vi "Load Config.vi"(10 "Cluster":T1, 11 "Process":bool) -> ()   [LabVIEW 2016]
uses:
  <vilib>/Utility/config.llb/Read Key (Double).vi
  <vilib>/Utility/config.llb/Read Key (Boolean).vi
  <vilib>/Utility/config.llb/NI_LVConfig.lvlib
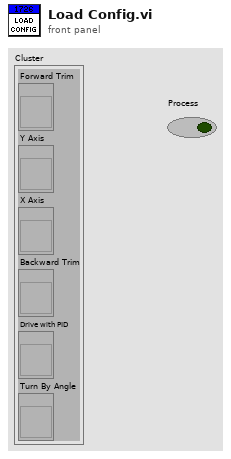
[diagram p1: front panel]
types:
  T1 = cluster{"Forward Trim":refnum<vi>, "Y Axis":refnum<vi>, "X Axis":refnum<vi>, "Backward Trim":refnum<vi>, "Drive with PID":refnum<vi>, "Turn By Angle":refnum<vi>}
  T2 = typedef "NI_LVConfig.lvlib/Config Data RefNum.ctl" = refnum<k1>
  T3 = cluster{"value":dbl, "value":dbl, "value":dbl, "value":bool}
  T4 = cluster{"value":dbl, dbl[], "value":dbl, "value":dbl}
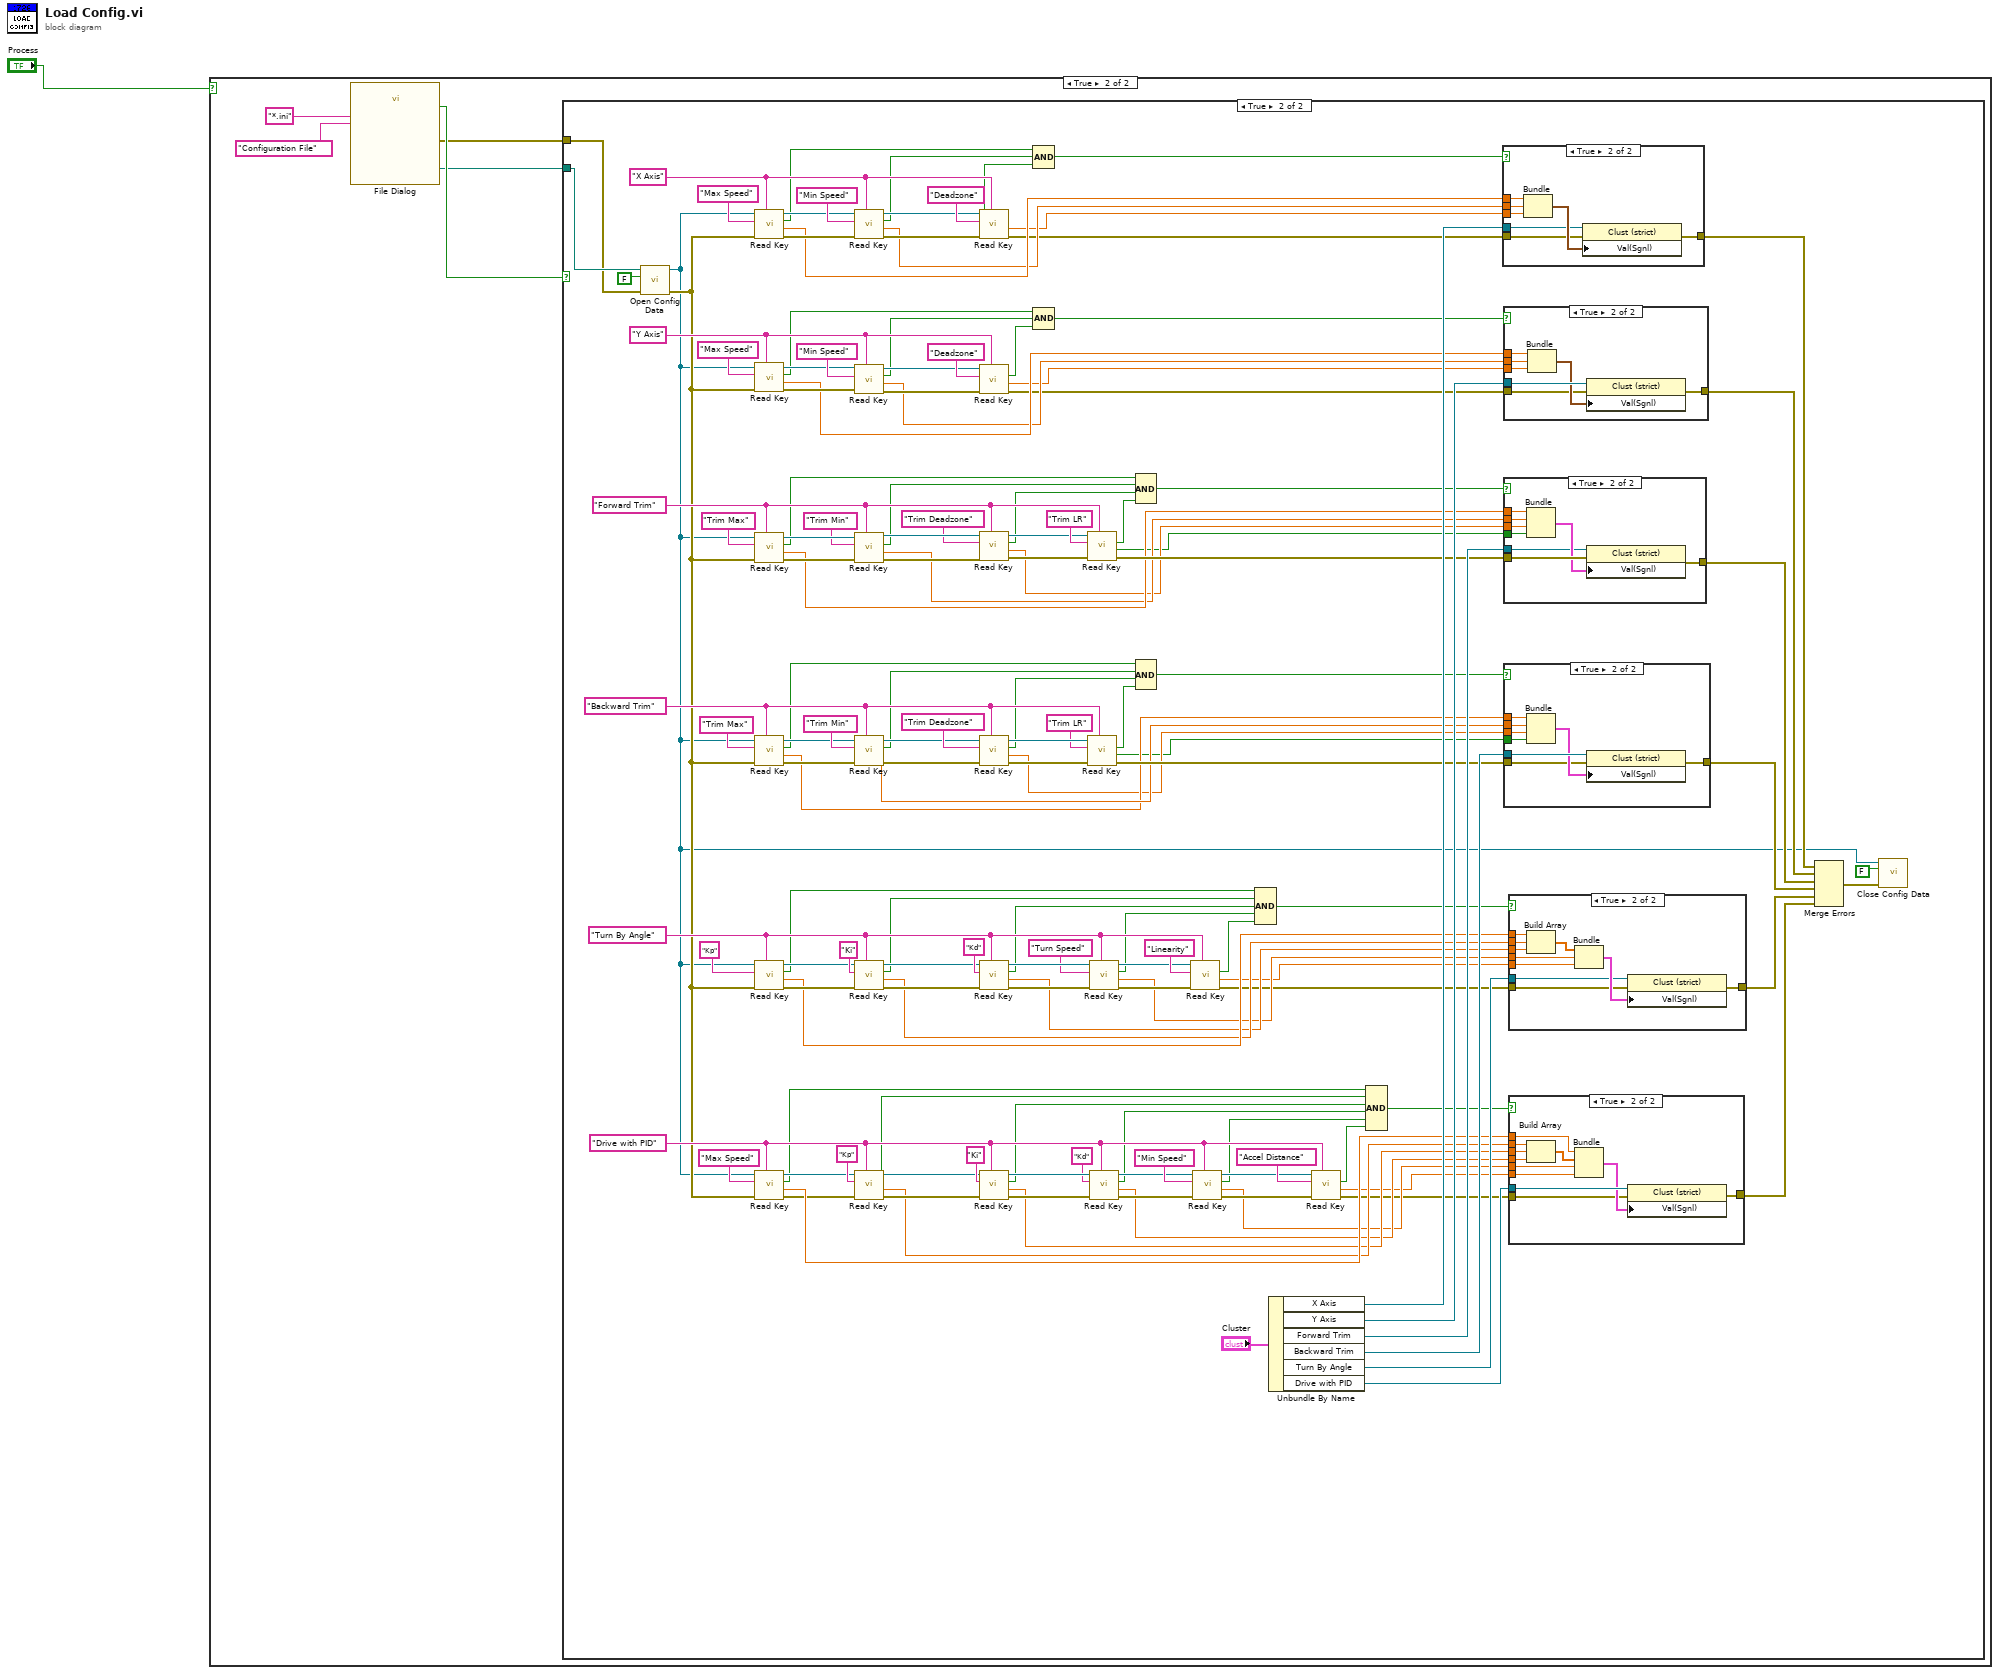
[diagram p0: block diagram]
diagram:
  n1 = case shown="True" "Process" {
    frame False {
    }
    frame True {
      n2 = call "File Dialog"("pattern (all files)"="*.ini", "pattern label"="Configuration File") -> ("selected path"=w3:path, "exists"=w4:bool, "error out"=w2:errorcluster)  [unwired: 10 in, 1 out]
      n3 = case shown="True" w4 {
        tunnel: w3 -> [_ w141]
        tunnel: w2 -> [_ w139]
        frame False {
        }
        frame True {
          w32 = "Drive with PID" ("section")
          w60 = "Turn By Angle" ("section")
          w83 = "Backward Trim" ("section")
          w118 = "Forward Trim" ("section")
          w134 = "Y Axis" ("section")
          w149 = "X Axis" ("section")
          n4 = call <vilib>:"Open Config Data.vi"("error in (no error)"=w139, "create file if necessary (T)"=FALSE, "configuration file path"=w141) -> ("error out"=w11:errorcluster, "refnum"=w8:T2)  [unwired: 6 in, 1 out]
          n5 = call-poly <vilib>:"Read Key.vi"("section"=w149, "error in (no error)"=w11, "key"="Max Speed", "refnum"=w8) -> ("error out"=w148:errorcluster, "value"=w138:dbl, "found?"=w111:bool, "refnum out"=w143:T2)  [unwired: 4 in]
          n6 = call-poly <vilib>:"Read Key.vi"("section"=w134, "error in (no error)"=w11, "key"="Max Speed", "refnum"=w8) -> ("error out"=w128:errorcluster, "value"=w126:dbl, "found?"=w107:bool, "refnum out"=w131:T2)  [unwired: 4 in]
          n7 = call-poly <vilib>:"Read Key.vi"("section"=w118, "error in (no error)"=w11, "key"="Trim Max", "refnum"=w8) -> ("error out"=w112:errorcluster, "value"=w97:dbl, "found?"=w103:bool, "refnum out"=w116:T2)  [unwired: 4 in]
          n8 = call-poly <vilib>:"Read Key.vi"("section"=w83, "error in (no error)"=w11, "key"="Trim Max", "refnum"=w8) -> ("error out"=w93:errorcluster, "value"=w75:dbl, "found?"=w82:bool, "refnum out"=w89:T2)  [unwired: 4 in]
          n9 = call-poly <vilib>:"Read Key.vi"("section"=w60, "error in (no error)"=w11, "key"="Kp", "refnum"=w8) -> ("error out"=w72:errorcluster, "value"=w52:dbl, "found?"=w58:bool, "refnum out"=w68:T2)  [unwired: 4 in]
          n10 = call-poly <vilib>:"Read Key.vi"("section"=w32, "error in (no error)"=w11, "key"="Max Speed", "refnum"=w8) -> ("error out"=w46:errorcluster, "value"=w151:dbl, "found?"=w29:bool, "refnum out"=w42:T2)  [unwired: 4 in]
          n11 = call-poly <vilib>:"Read Key.vi"("section"=w149, "error in (no error)"=w148, "key"="Min Speed", "refnum"=w143) -> ("error out"=w147:errorcluster, "value"=w137:dbl, "found?"=w110:bool, "refnum out"=w142:T2)  [unwired: 4 in]
          n12 = call-poly <vilib>:"Read Key.vi"("section"=w134, "error in (no error)"=w128, "key"="Min Speed", "refnum"=w131) -> ("error out"=w127:errorcluster, "value"=w125:dbl, "found?"=w106:bool, "refnum out"=w130:T2)  [unwired: 4 in]
          n13 = call-poly <vilib>:"Read Key.vi"("section"=w118, "error in (no error)"=w112, "key"="Trim Min", "refnum"=w116) -> ("error out"=w113:errorcluster, "value"=w96:dbl, "found?"=w102:bool, "refnum out"=w117:T2)  [unwired: 4 in]
          n14 = call-poly <vilib>:"Read Key.vi"("section"=w83, "error in (no error)"=w93, "key"="Trim Min", "refnum"=w89) -> ("error out"=w92:errorcluster, "value"=w76:dbl, "found?"=w81:bool, "refnum out"=w88:T2)  [unwired: 4 in]
          n15 = call-poly <vilib>:"Read Key.vi"("section"=w60, "error in (no error)"=w72, "key"="Ki", "refnum"=w68) -> ("error out"=w71:errorcluster, "value"=w51:dbl, "found?"=w57:bool, "refnum out"=w67:T2)  [unwired: 4 in]
          n16 = call-poly <vilib>:"Read Key.vi"("section"=w32, "error in (no error)"=w46, "key"="Kp", "refnum"=w42) -> ("error out"=w45:errorcluster, "value"=w23:dbl, "found?"=w28:bool, "refnum out"=w41:T2)  [unwired: 4 in]
          n17 = call-poly <vilib>:"Read Key.vi"("section"=w149, "error in (no error)"=w147, "key"="Deadzone", "refnum"=w142) -> ("error out"=w135:errorcluster, "value"=w136:dbl, "found?"=w109:bool)  [unwired: 4 in, 1 out]
          n18 = call-poly <vilib>:"Read Key.vi"("section"=w134, "error in (no error)"=w127, "key"="Deadzone", "refnum"=w130) -> ("error out"=w123:errorcluster, "value"=w124:dbl, "found?"=w105:bool)  [unwired: 4 in, 1 out]
          n19 = call-poly <vilib>:"Read Key.vi"("section"=w118, "error in (no error)"=w113, "key"="Trim Deadzone", "refnum"=w117) -> ("error out"=w119:errorcluster, "value"=w95:dbl, "found?"=w101:bool, "refnum out"=w120:T2)  [unwired: 4 in]
          n20 = call-poly <vilib>:"Read Key.vi"("section"=w83, "error in (no error)"=w92, "key"="Trim Deadzone", "refnum"=w88) -> ("error out"=w87:errorcluster, "value"=w74:dbl, "found?"=w80:bool, "refnum out"=w86:T2)  [unwired: 4 in]
          n21 = call-poly <vilib>:"Read Key.vi"("section"=w60, "error in (no error)"=w71, "key"="Kd", "refnum"=w67) -> ("error out"=w66:errorcluster, "value"=w50:dbl, "found?"=w56:bool, "refnum out"=w65:T2)  [unwired: 4 in]
          n22 = call-poly <vilib>:"Read Key.vi"("section"=w32, "error in (no error)"=w45, "key"="Ki", "refnum"=w41) -> ("error out"=w40:errorcluster, "value"=w22:dbl, "found?"=w27:bool, "refnum out"=w39:T2)  [unwired: 4 in]
          n23 = Compound Arithmetic op=AND(w111, w110, w109) -> (w108:bool)
          n24 = Compound Arithmetic op=AND(w107, w106, w105) -> (w104:bool)
          n25 = call-poly <vilib>:"Read Key.vi"("section"=w118, "error in (no error)"=w119, "key"="Trim LR", "refnum"=w120) -> ("error out"=w98:errorcluster, "value"=w94:bool, "found?"=w100:bool)  [unwired: 4 in, 1 out]
          n26 = call-poly <vilib>:"Read Key.vi"("section"=w83, "error in (no error)"=w87, "key"="Trim LR", "refnum"=w86) -> ("error out"=w78:errorcluster, "value"=w73:bool, "found?"=w79:bool)  [unwired: 4 in, 1 out]
          n27 = call-poly <vilib>:"Read Key.vi"("section"=w60, "error in (no error)"=w66, "key"="Turn Speed", "refnum"=w65) -> ("error out"=w61:errorcluster, "value"=w49:dbl, "found?"=w55:bool, "refnum out"=w59:T2)  [unwired: 4 in]
          n28 = call-poly <vilib>:"Read Key.vi"("section"=w32, "error in (no error)"=w40, "key"="Kd", "refnum"=w39) -> ("error out"=w34:errorcluster, "value"=w21:dbl, "found?"=w26:bool, "refnum out"=w31:T2)  [unwired: 4 in]
          n29 = Compound Arithmetic op=AND(w103, w102, w101, w100) -> (w99:bool)
          n30 = Compound Arithmetic op=AND(w82, w81, w80, w79) -> (w77:bool)
          n31 = call-poly <vilib>:"Read Key.vi"("section"=w60, "error in (no error)"=w61, "key"="Linearity", "refnum"=w59) -> ("error out"=w47:errorcluster, "value"=w48:dbl, "found?"=w54:bool)  [unwired: 4 in, 1 out]
          n32 = call-poly <vilib>:"Read Key.vi"("section"=w32, "error in (no error)"=w34, "key"="Min Speed", "refnum"=w31) -> ("error out"=w33:errorcluster, "value"=w20:dbl, "found?"=w25:bool, "refnum out"=w30:T2)  [unwired: 4 in]
          n33 = Compound Arithmetic op=AND(w58, w57, w56, w55, w54) -> (w53:bool)
          n34 = Unbundle By Name("Cluster") -> ("X Axis"=w154:refnum<vi>, "Y Axis"=w157:refnum<vi>, "Forward Trim"=w155:refnum<vi>, "Backward Trim"=w156:refnum<vi>, "Turn By Angle"=w153:refnum<vi>, "Drive with PID"=w152:refnum<vi>)
          n35 = call-poly <vilib>:"Read Key.vi"("section"=w32, "error in (no error)"=w33, "key"="Accel Distance", "refnum"=w30) -> ("error out"=w18:errorcluster, "value"=w19:dbl, "found?"=w24:bool)  [unwired: 4 in, 1 out]
          n36 = Compound Arithmetic op=AND(w29, w28, w27, w26, w25, w24) -> (w7:bool)
          n37 = case shown="True" w108 {
            tunnel: w138 -> [_ w214]
            tunnel: w137 -> [_ w213]
            tunnel: w136 -> [_ w212]
            tunnel: w154 -> [_ w210]
            tunnel: w135 -> [w207 w209]
            tunnel: [w207 w208] -> w17
            frame False {
            }
            frame True {
              n38 = Bundle("value"=w214, "value"=w213, "value"=w212) -> (w211:cluster{"value":dbl, "value":dbl, "value":dbl})  [unwired: 1 in]
              n39 = property class="Clust (strict)"(reference=w210, error in=w209, "Val(Sgnl)"=w211) -> (error out=w208:errorcluster)  [unwired: 1 out]
            }
          }
          n40 = case shown="True" w104 {
            tunnel: w157 -> [_ w206]
            tunnel: w126 -> [_ w205]
            tunnel: w125 -> [_ w204]
            tunnel: w124 -> [_ w203]
            tunnel: w123 -> [w199 w201]
            tunnel: [w199 w200] -> w16
            frame False {
            }
            frame True {
              n41 = Bundle("value"=w205, "value"=w204, "value"=w203) -> (w202:cluster{"value":dbl, "value":dbl, "value":dbl})  [unwired: 1 in]
              n42 = property class="Clust (strict)"(reference=w206, error in=w201, "Val(Sgnl)"=w202) -> (error out=w200:errorcluster)  [unwired: 1 out]
            }
          }
          n43 = case shown="True" w99 {
            tunnel: w98 -> [w190 w194]
            tunnel: w97 -> [_ w198]
            tunnel: w96 -> [_ w197]
            tunnel: w95 -> [_ w196]
            tunnel: w94 -> [_ w195]
            tunnel: [w190 w193] -> w15
            tunnel: w155 -> [_ w191]
            frame False {
            }
            frame True {
              n44 = Bundle("value"=w198, "value"=w197, "value"=w196, "value"=w195) -> (w192:T3)  [unwired: 1 in]
              n45 = property class="Clust (strict)"(reference=w191, error in=w194, "Val(Sgnl)"=w192) -> (error out=w193:errorcluster)  [unwired: 1 out]
            }
          }
          n46 = case shown="True" w77 {
            tunnel: w78 -> [w181 w182]
            tunnel: w76 -> [_ w189]
            tunnel: w75 -> [_ w188]
            tunnel: w74 -> [_ w187]
            tunnel: w73 -> [_ w186]
            tunnel: w156 -> [_ w185]
            tunnel: [w181 w183] -> w14
            frame False {
            }
            frame True {
              n47 = Bundle("value"=w188, "value"=w189, "value"=w187, "value"=w186) -> (w184:T3)  [unwired: 1 in]
              n48 = property class="Clust (strict)"(reference=w185, error in=w182, "Val(Sgnl)"=w184) -> (error out=w183:errorcluster)  [unwired: 1 out]
            }
          }
          n49 = case shown="True" w53 {
            tunnel: w52 -> [_ w180]
            tunnel: w51 -> [_ w179]
            tunnel: w50 -> [_ w178]
            tunnel: w49 -> [_ w176]
            tunnel: w48 -> [_ w175]
            tunnel: w153 -> [_ w173]
            tunnel: w47 -> [w170 w172]
            tunnel: [w170 w171] -> w13
            frame False {
            }
            frame True {
              n50 = Build Array(w180, w179, w178) -> (w177:dbl[])
              n51 = Bundle(w177, "value"=w176, "value"=w175) -> (w174:cluster{dbl[], "value":dbl, "value":dbl})  [unwired: 1 in]
              n52 = property class="Clust (strict)"(reference=w173, error in=w172, "Val(Sgnl)"=w174) -> (error out=w171:errorcluster)  [unwired: 1 out]
            }
          }
          n53 = case shown="True" w7 {
            tunnel: w23 -> [_ w169]
            tunnel: w22 -> [_ w168]
            tunnel: w21 -> [_ w167]
            tunnel: w151 -> [_ w165]
            tunnel: w20 -> [_ w164]
            tunnel: w19 -> [_ w163]
            tunnel: w152 -> [_ w162]
            tunnel: w18 -> [w158 w160]
            tunnel: [w158 w159] -> w12
            frame False {
            }
            frame True {
              n54 = Build Array(w169, w168, w167) -> (w166:dbl[])
              n55 = Bundle("value"=w165, w166, "value"=w164, "value"=w163) -> (w161:T4)  [unwired: 1 in]
              n56 = property class="Clust (strict)"(reference=w162, error in=w160, "Val(Sgnl)"=w161) -> (error out=w159:errorcluster)  [unwired: 1 out]
            }
          }
          n57 = Merge Errors(w17, w16, w15, w14, w13, w12) -> (w10:errorcluster)
          n58 = call <vilib>:"Close Config Data.vi"("error in (no error)"=w10, "write file if changed (T)"=FALSE, "refnum"=w8) -> ()  [unwired: 7 in, 2 out]
        }
      }
    }
  }
